vi "Read Spreadsheet File.vi"(6 "Delimiter (tab)":string="\t", 8 "error in (no error)":errorcluster, 11 "File Path":path) -> (0 "error out":errorcluster, 3 "2D Array":string[][](array[string]))   [LabVIEW 2016, in "SLL Spreadsheet.lvlib"]
doc: "Reads a spreadsheet file and returns 2D string array, similar to how Excel does when any cells contain new line character, comma or quotes."
uses:
  SLL Spreadsheet.lvlib
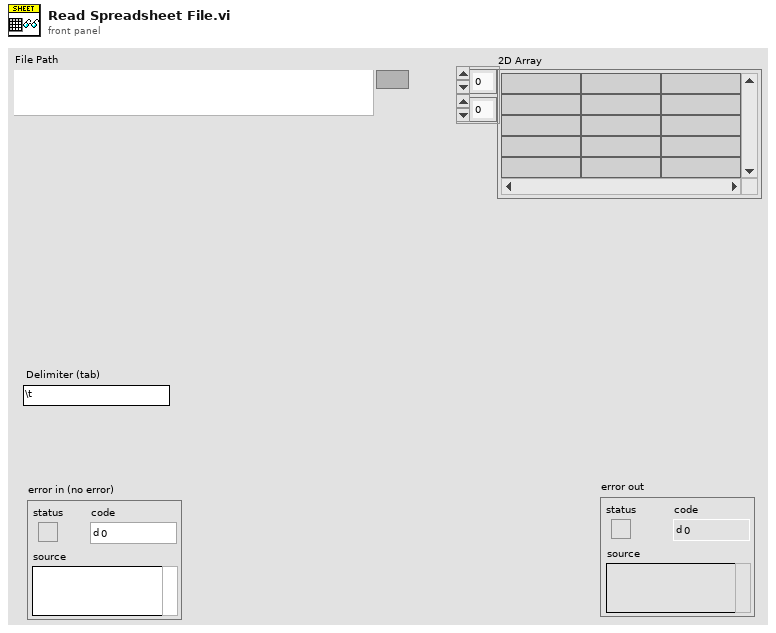
[diagram p1: front panel]
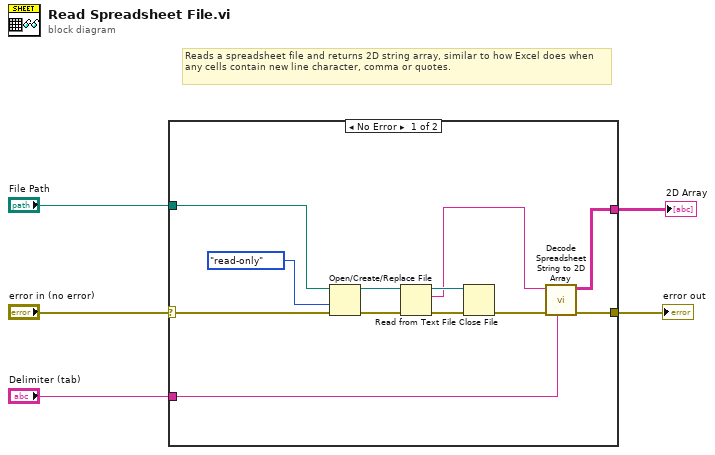
[diagram p0: block diagram]
diagram:
  # "Reads a spreadsheet file and returns 2D string array, similar to how Excel does when any cells contain new line character, comma or quotes."
  n1 = case shown="No Error" "error in (no error)" {
    selector: "error in (no error)" -> [w14 w18]
    tunnel: "File Path" -> [w15 _]
    tunnel: [w9 w18] -> w3
    tunnel: "Delimiter (tab)" -> [w7 _]
    tunnel: [w6 _] -> w1
    frame No Error {
      n2 = Open/Create/Replace File(file path (use dialog)=w15, error in=w14, access (0:read/write)=enum16{"read/write", "read-only", "write-only"}."read-only") -> (refnum out=w12:refnum<file>, error out=w13:errorcluster)  [unwired: 3 in, 1 out]
      n3 = Read from Text File(file (use dialog)=w12, error in=w13) -> (refnum out=w17:refnum<file>, text=w8:string, error out=w16:errorcluster)  [unwired: 2 in, 1 out]
      n4 = Close File(refnum=w17, error in=w16) -> (error out=w10:errorcluster)  [unwired: 1 out]
      n5 = call "Decode Spreadsheet String to 2D Array.vi"("Delimiter (,)"=w7, "error in (no error)"=w10, "Spreadsheet String"=w8) -> ("error out"=w9:errorcluster, "2D Array"=w6:string[][])  [unwired: 7 in]
    }
    frame Error {
    }
  }
  "error out" <- w3
  "2D Array" <- w1
